vi "REG - Display2DTest.vi"(8 "error in":errorcluster, 11 "Local":T5={"Parameters"={"Plot"=refnum, "Data"={"Split"={"X Train"=[], "X Test"=[], "Y Train"=[], "Y Test"=[]}, "Predict"=[]}, "Display"={"Choice"=enum."All", "Indexe"={"X"=0, "Y"=1}}, "Point Property"={"Train Style"=enum."Full circle", "Test OK Style"=enum."Full square", "Label Color"=[8978528, 4367871, 16716800], "Test NO OK"={"Style"=enum."Cross", "Color"=16711680}}, "Tolerance's threshold"=0.0}, "2D Array"=[], "Point ID"=[], "GoodPredict"=0, "Rating 2D Array"=[]}) -> (0 "error out":errorcluster, 3 "Local Out":T5={"Parameters"={"Plot"=refnum, "Data"={"Split"={"X Train"=[], "X Test"=[], "Y Train"=[], "Y Test"=[]}, "Predict"=[]}, "Display"={"Choice"=enum."All", "Indexe"={"X"=0, "Y"=1}}, "Point Property"={"Train Style"=enum."Full circle", "Test OK Style"=enum."Full square", "Label Color"=[8978528, 4367871, 16716800], "Test NO OK"={"Style"=enum."Cross", "Color"=16711680}}, "Tolerance's threshold"=0.0}, "2D Array"=[], "Point ID"=[], "GoodPredict"=0, "Rating 2D Array"=[]})   [LabVIEW 2020]
uses:
  _Controls/Datas.ctl
  _Controls/PointPropertyMultipleLabel.ctl
  _Controls/Style.ctl
  _Controls/2DData.ctl
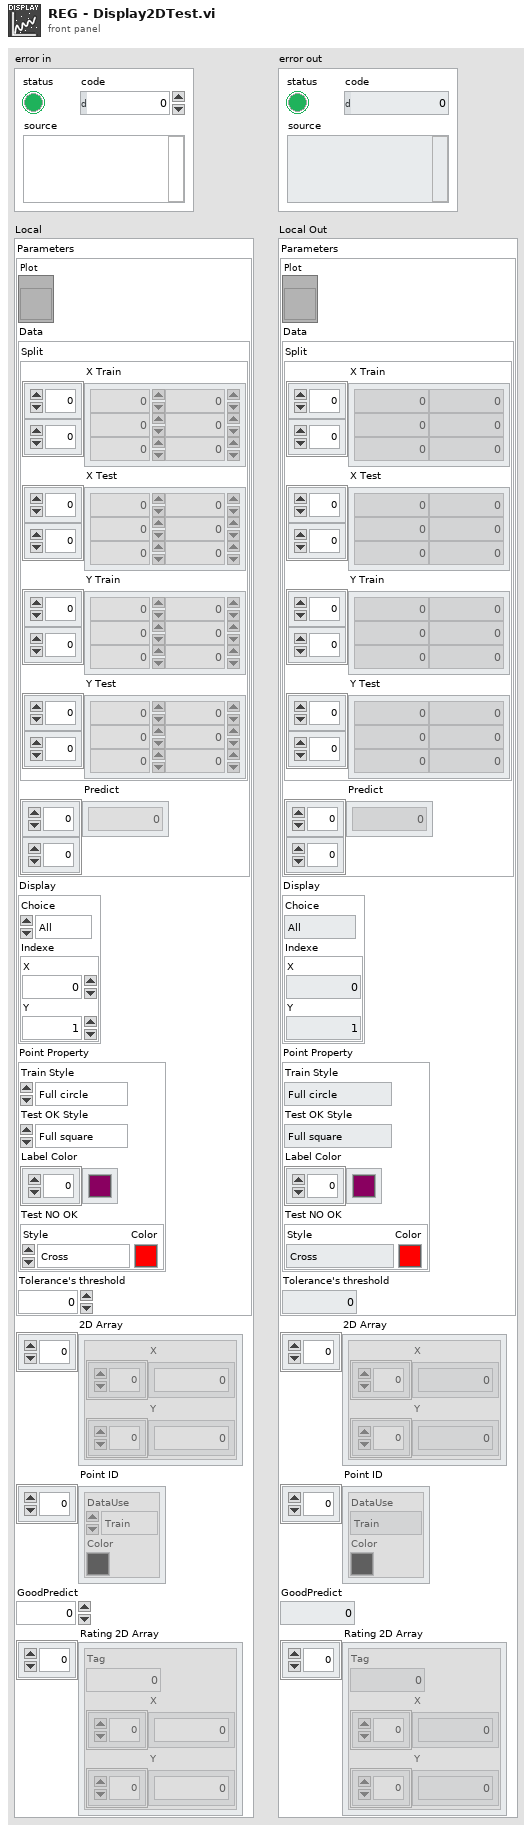
[diagram p1: front panel]
types:
  T1 = typedef "Datas.ctl" = cluster{"Split":cluster{"X Train":dbl[][], "X Test":dbl[][], "Y Train":dbl[][], "Y Test":dbl[][]}, "Predict":dbl[][]}
  T2 = typedef "PointPropertyMultipleLabel.ctl" = cluster{"Train Style":T3, "Test OK Style":T3, "Label Color":u32[], "Test NO OK":cluster{"Style":T3, "Color":u32}}
  T3 = typedef "Style.ctl" = enum16{"Empty circle", "Full circle", "Empty square", "Full square", "Cross"}
  T4 = typedef "2DData.ctl" = cluster{"Tag":i32, "X":dbl[], "Y":dbl[]}
  T5 = cluster{"Parameters":cluster{"Plot":refnum<vi>, "Data":T1, "Display":cluster{"Choice":enum16{"All", "Train", "Test"}, "Indexe":cluster{"X":i32, "Y":i32}}, "Point Property":T2, "Tolerance's threshold":dbl}, "2D Array":cluster{"X":dbl[], "Y":dbl[]}[], "Point ID":cluster{"DataUse":enum16{"Dataset", "Train", "Test"}, "Color":u32}[], "GoodPredict":i32, "Rating 2D Array":T4[]}
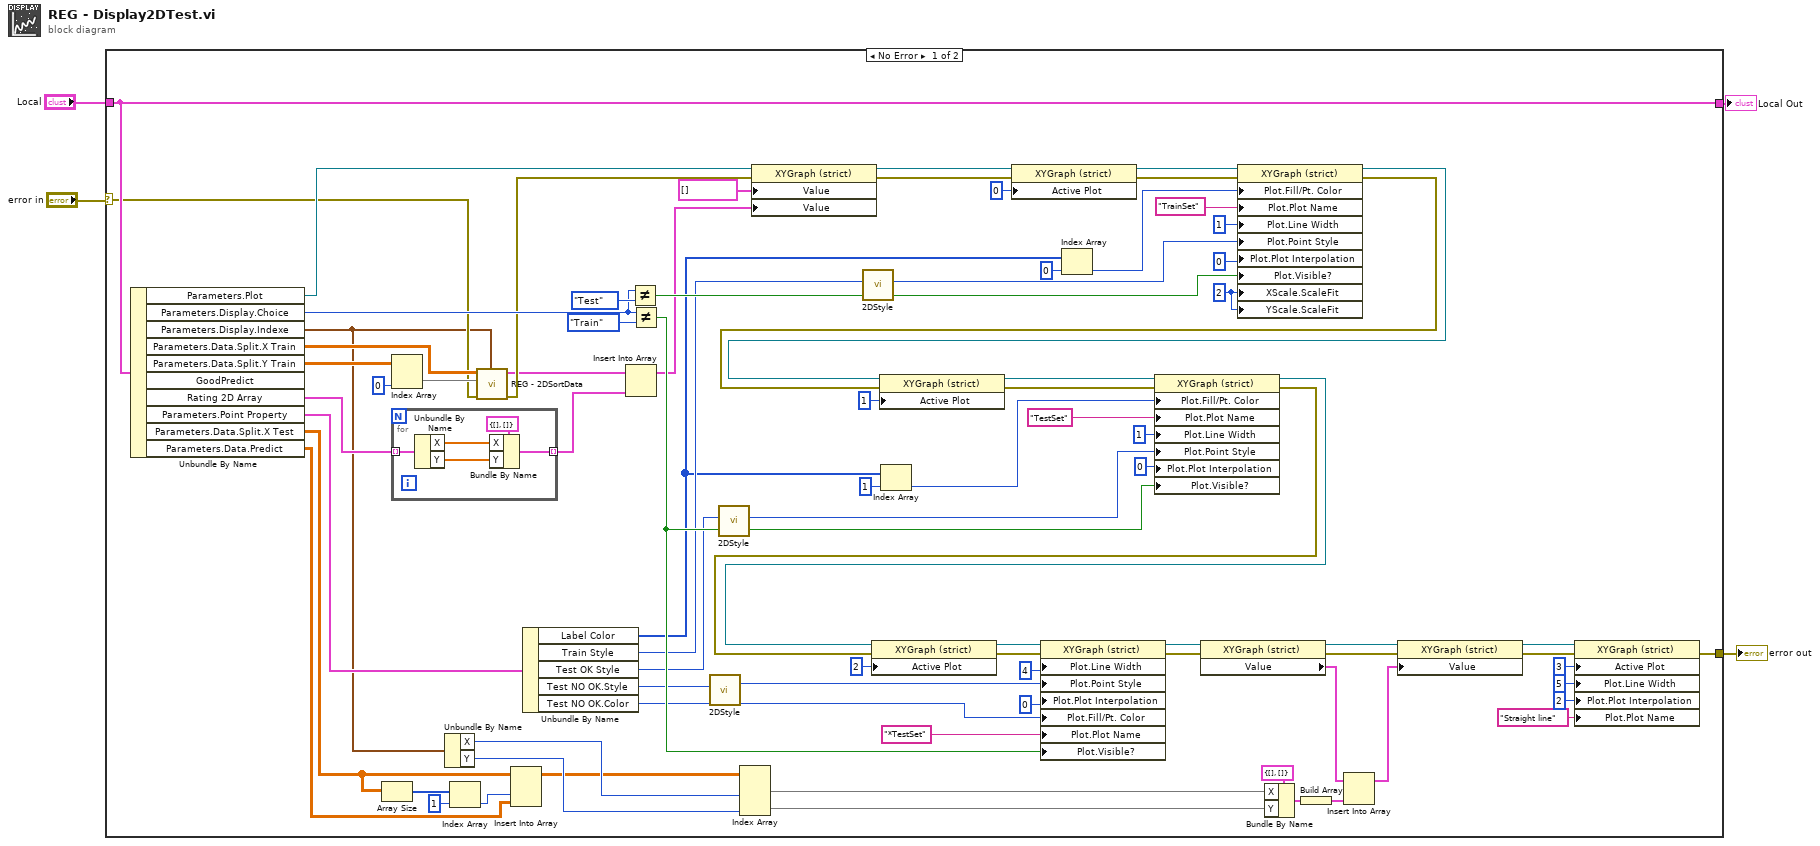
[diagram p0: block diagram]
diagram:
  n1 = case shown="No Error" "error in" {
    selector: "error in" -> [w48 w94]
    tunnel: [w53 w94] -> w3
    tunnel: "Local" -> [w73 w93]
    tunnel: [w73 w93] -> w1
    frame No Error {
      w30 = u8 2 ("X Scale.Scale Fit")
      n2 = Unbundle By Name(w73) -> ("Parameters.Plot"=w76:refnum<vi>, "Parameters.Display.Choice"=w72:enum16{"All", "Train", "Test"}, "Parameters.Display.Indexe"=w16:cluster{"X":i32, "Y":i32}, "Parameters.Data.Split.X Train"=w50:dbl[][], "Parameters.Data.Split.Y Train"=w77:dbl[][], "Rating 2D Array"=w79:T4[], "Parameters.Point Property"=w68:T2, "Parameters.Data.Split.X Test"=w9:dbl[][], "Parameters.Data.Predict"=w10:dbl[][])  [unwired: 1 out]
      n3 = Array Size(array=w9) -> (size(s)=w8:i32[])
      n4 = Index Array(array=w77, index (col)=0 ("disabled index (col)")) -> (element=w49:dbl[])  [unwired: 1 in]
      n5 = for {
        tunnel: w79 -> [w92] mode=indexing
        tunnel: [w88] -> w83 mode=indexing
        n6 = Unbundle By Name(w92) -> ("X"=w90:dbl[], "Y"=w89:dbl[])
        n7 = Bundle By Name(cluster=cluster{"X":dbl[], "Y":dbl[]} {"X"=[], "Y"=[]} ("new element/subarray"), "X"=w90, "Y"=w89) -> (w88:cluster{"X":dbl[], "Y":dbl[]})
      }
      n8 = Unbundle By Name(w16) -> ("X"=w15:i32, "Y"=w14:i32)
      n9 = Index Array(array=w8, index=1) -> (element=w6:i32)
      n10 = call "REG - 2DSortData.vi"("Index"=w16, "error in"=w48, "Y"=w49, "X"=w50) -> ("error out"=w51:errorcluster, "Array"=w35:cluster{"Array":dbl[], "Array":dbl[]}[])  [unwired: 6 in]
      n11 = Insert Into Array(array=w9, index (col)=w6, new element=w10) -> (w11:dbl[][])  [unwired: 1 in]
      n12 = Unbundle By Name(w68) -> ("Label Color"=w18:u32[], "Train Style"=w66:T3, "Test OK Style"=w64:T3, "Test NO OK.Style"=w62:T3, "Test NO OK.Color"=w67:u32)
      n13 = Insert Into Array(array=w35, new element=w83) -> (w71:cluster{"Array":dbl[], "Array":dbl[]}[])  [unwired: 1 in]
      n14 = Not Equal?(x=w72, y=enum16{"All", "Train", "Test"}."Test") -> (x != y?=w81:bool)
      n15 = Not Equal?(x=w72, y=enum16{"All", "Train", "Test"}."Train") -> (x != y?=w80:bool)
      n16 = call "2DStyle.vi"("Style"=w62) -> ("Style"=w61:u8)  [unwired: 10 in]
      n17 = call "2DStyle.vi"("Style"=w64) -> ("Style"=w63:u8)  [unwired: 10 in]
      n18 = Index Array(array=w11, index (col) #1=w15, index (col) #2=w14) -> (element #1=w13:dbl[], element #2=w12:dbl[])  [unwired: 2 in]
      n19 = property class="XYGraph (strict)"(reference=w76, error in=w51, "Value"=cluster{"X":dbl[], "Y":dbl[]}[] [], "Value"=w71) -> (reference out=w75:refnum<vi>, error out=w74:errorcluster)
      n20 = call "2DStyle.vi"("Style"=w66) -> ("Style"=w65:u8)  [unwired: 10 in]
      n21 = Index Array(array=w18, index=1) -> (element=w17:u32)
      n22 = property class="XYGraph (strict)"(reference=w75, error in=w74, "Active Plot"=u32 0) -> (reference out=w34:refnum<vi>, error out=w33:errorcluster)
      n23 = Index Array(array=w18, index=0) -> (element=w27:u32)
      n24 = property class="XYGraph (strict)"(reference=w34, error in=w33, "Plot.Fill/Pt. Color"=w27, "Plot.Plot Name"="TrainSet", "Plot.Line Width"=u8 1, "Plot.Point Style"=w65, "Plot.Plot Interpolation"=u8 0, "Plot.Visible?"=w81, "XScale.ScaleFit"=w30, "YScale.ScaleFit"=w30) -> (reference out=w86:refnum<vi>, error out=w87:errorcluster)
      n25 = property class="XYGraph (strict)"(reference=w86, error in=w87, "Active Plot"=u32 1) -> (reference out=w22:refnum<vi>, error out=w21:errorcluster)
      n26 = property class="XYGraph (strict)"(reference=w22, error in=w21, "Plot.Fill/Pt. Color"=w17, "Plot.Plot Name"="TestSet", "Plot.Line Width"=u8 1, "Plot.Point Style"=w63, "Plot.Plot Interpolation"=u8 0, "Plot.Visible?"=w80) -> (reference out=w85:refnum<vi>, error out=w84:errorcluster)
      n27 = property class="XYGraph (strict)"(reference=w85, error in=w84, "Active Plot"=u32 2) -> (reference out=w60:refnum<vi>, error out=w59:errorcluster)
      n28 = property class="XYGraph (strict)"(reference=w60, error in=w59, "Plot.Line Width"=u8 4, "Plot.Point Style"=w61, "Plot.Plot Interpolation"=u8 0, "Plot.Fill/Pt. Color"=w67, "Plot.Plot Name"="*TestSet", "Plot.Visible?"=w80) -> (reference out=w54:refnum<vi>, error out=w55:errorcluster)
      n29 = property class="XYGraph (strict)"(reference=w54, error in=w55) -> (reference out=w44:refnum<vi>, error out=w45:errorcluster, "Value"=w46:cluster{"X":dbl[], "Y":dbl[]}[])
      n30 = Bundle By Name(cluster=cluster{"X":dbl[], "Y":dbl[]} {"X"=[], "Y"=[]} ("new element/subarray"), "X"=w13, "Y"=w12) -> (w37:cluster{"X":dbl[], "Y":dbl[]})
      n31 = Build Array(w37) -> (w36:cluster{"X":dbl[], "Y":dbl[]}[])
      n32 = Insert Into Array(array=w46, new element=w36) -> (w43:cluster{"X":dbl[], "Y":dbl[]}[])  [unwired: 1 in]
      n33 = property class="XYGraph (strict)"(reference=w44, error in=w45, "Value"=w43) -> (reference out=w5:refnum<vi>, error out=w42:errorcluster)
      n34 = property class="XYGraph (strict)"(reference=w5, error in=w42, "Active Plot"=u32 3, "Plot.Line Width"=u8 5, "Plot.Plot Interpolation"=u8 2, "Plot.Plot Name"="Straight line") -> (error out=w53:errorcluster)  [unwired: 1 out]
    }
    frame Error {
    }
  }
  "error out" <- w3
  "Local Out" <- w1
